vi "ABC Find Close - Bladder.vi"(4 "UART":refnum<vi>, 5 "ComPort":refnum<visa-resource-name>, 6 "Data":refnum<vi>, 7 "DaqTask":refnum<k21>, 8 "ErrIn":errorcluster, 11 "DataIn":dbl[](array[numeric])=[0.0]) -> (0 "ErrOut":errorcluster, 1 "BlaPos":dbl, 3 "DataOut":dbl[](array[numeric]))   [LabVIEW 2020]
uses:
  <vilib>/DAQmx/read.llb/DAQmx Read (Digital 1D Bool 1Chan 1Samp).vi
  <vilib>/DAQmx/miscellaneous.llb/DAQmx Fill In Error Info.vi
  <userlib>/KQD LabVIEW User/Serial/Serial.lvlib
panel:
  out "BladderSW":bool
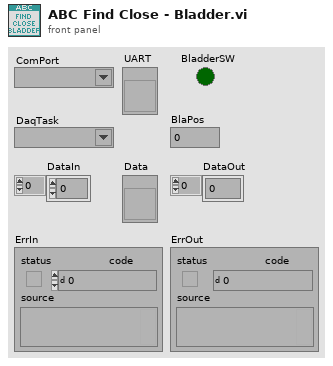
[diagram p1: front panel]
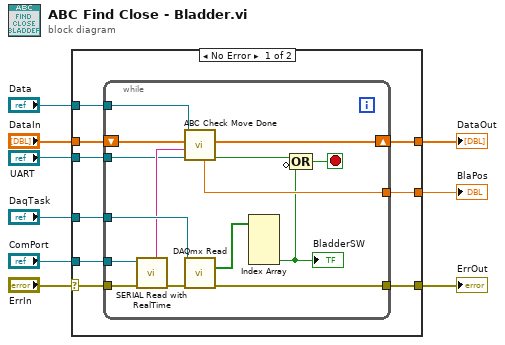
[diagram p0: block diagram]
diagram:
  n1 = case shown="No Error" "ErrIn" {
    selector: "ErrIn" -> [w11 w34]
    tunnel: "UART" -> [w13 _]
    tunnel: "DaqTask" -> [w18 _]
    tunnel: [w17 w34] -> w7
    tunnel: "DataIn" -> [w16 w35]
    tunnel: [w15 w35] -> w5
    tunnel: "ComPort" -> [w14 _]
    tunnel: "Data" -> [w12 _]
    tunnel: [w10 _] -> w1
    frame No Error {
      n2 = while {
        tunnel: w18 -> [w32]
        tunnel: w12 -> [w27]
        tunnel: w14 -> [w31]
        shift-right: [w24] -> w15
        shift-left: w16 -> [w28]
        tunnel: [w29] -> w17
        tunnel: w13 -> [w25]
        tunnel: w11 -> [w21]
        tunnel: [w20] -> w10
        stop <- w23 stop-if-true
        n3 = call <userlib>:"SERIAL Read with RealTime.vi"("ErrIn"=w21, "PortIn"=w31) -> ("ErrOut"=w30:errorcluster, "Response"=w26:string)  [unwired: 7 in, 1 out]
        n4 = call "ABC Check Move Done.vi"("UART"=w25, "Response"=w26, "DataIn"=w28, "Data"=w27) -> ("Done"=w22:bool, "DataOut"=w24:dbl[], "Position"=w20:dbl)  [unwired: 5 in]
        n5 = call-poly <vilib>:"DAQmx Read.vi"("task/channels in"=w32, "error in"=w30) -> ("data"=w33:bool[], "error out"=w29:errorcluster)  [unwired: 11 in, 1 out]
        n6 = Index Array(array=w33) -> (element #4=w19:bool)  [unwired: 4 in, 3 out]
        "BladderSW" <- w19
        n7 = Compound Arithmetic op=OR(w22, invert w19) -> (w23:bool)
      }
    }
    frame Error {
    }
  }
  "ErrOut" <- w7
  "DataOut" <- w5
  "BlaPos" <- w1
